vi "Where.vi"(8 "error in (no error)":errorcluster, 11 "SQL Server in":refnum<class "SQL Server.lvclass">) -> (0 "error out":errorcluster, 3 "SQL Server out":refnum<class "SQL Server.lvclass">)   [LabVIEW 2021, in "SQL Server.lvclass"]
uses:
  <userlib>/John_Lib/DataBase/SQL Server/SQL Server.lvclass
  <userlib>/John_Lib/DataBase/SQL Server/SQL Server.lvclass/SQL Server.ctl
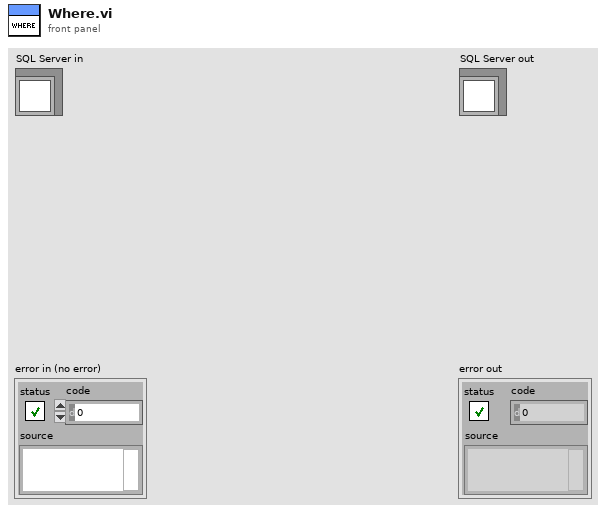
[diagram p1: front panel]
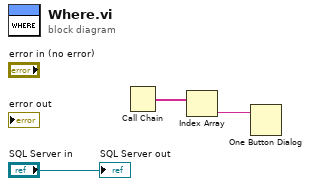
[diagram p0: block diagram]
diagram:
  n1 = Call Chain() -> (call chain=w1:string[])
  n2 = Index Array(array=w1) -> (element=w2:string)  [unwired: 1 in]
  n3 = One Button Dialog(message=w2) -> ()  [unwired: 1 in, 1 out]
  "SQL Server out" <- "SQL Server in"
